vi "Motor conditions_subVI.vi"(0 "Target Angle (°)":dbl, 5 "Current Angle (°)":dbl, 7 "Solenoid ON/OFF":bool, 9 "Stop":bool, 11 "error in (no error)":errorcluster) -> (4 "Motor On/Off":bool, 6 "Motor FWD/RVS":bool, 8 "Solenoid ON/OFF":bool, 10 "STOP":bool, 15 "error out":errorcluster)   [LabVIEW 2017]
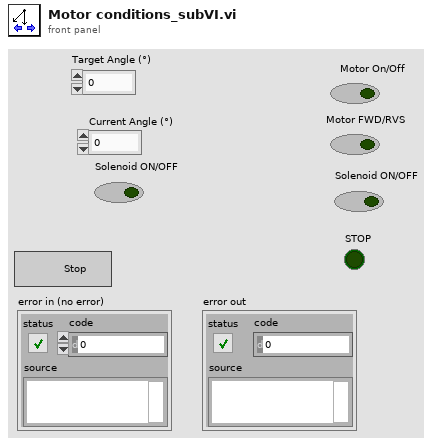
[diagram p1: front panel]
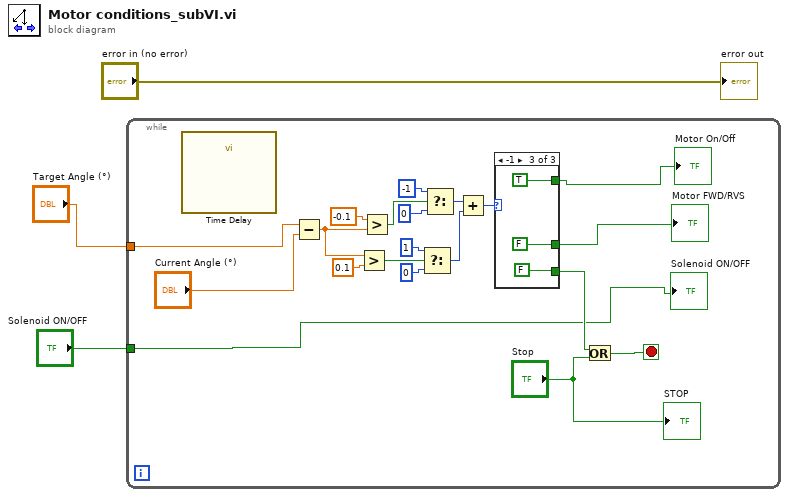
[diagram p0: block diagram]
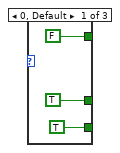
[diagram p2: hidden frame]
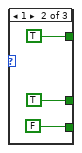
[diagram p3: hidden frame]
diagram:
  n1 = while {
    tunnel: "Target Angle (°)" -> [w9]
    tunnel: "Solenoid ON/OFF" -> [w4]
    stop <- w11 stop-if-true
    n2 = call "Time Delay"() -> ()  [unwired: 11 in, 1 out]
    n3 = Subtract(x=w9, y="Current Angle (°)") -> (x-y=w22:dbl)
    n4 = Greater?(x=w22, y=0.1) -> (0:w17:bool)
    n5 = Greater?(x=-0.1, y=w22) -> (0:w20:bool)
    n6 = Select(t=1, s=w17, f=0) -> (s? t:f=w13:i32)
    n7 = Select(t=-1, s=w20, f=0) -> (s? t:f=w14:i32)
    n8 = Add(x=w14, y=w13) -> (x+y=w12:i32)
    n9 = case shown="-1" w12 {
      tunnel: [TRUE TRUE FALSE] -> w7
      tunnel: [FALSE TRUE TRUE] -> w8
      tunnel: [TRUE FALSE FALSE] -> w10
      frame 0, Default {
      }
      frame 1 {
      }
      frame -1 {
      }
    }
    "Motor FWD/RVS" <- w7
    "Motor On/Off" <- w8
    n10 = Or(x=w10, y="Stop") -> (x .or. y?=w11:bool)
    "STOP" <- "Stop"
    "Solenoid ON/OFF" <- w4
  }
  "error out" <- "error in (no error)"
